vi "Verify Node GUID Matches Data Sharing Framework GUID.vi"(8 "error in":errorcluster, 11 "data sharing framework custom device in":T1 format="%.0x") -> (0 "error out":errorcluster, 3 "data sharing framework custom device out":T1 format="%.0x")   [LabVIEW 2021, in "Data Sharing Framework Custom Device Scripting.lvlib"]
uses:
  Data Sharing Framework Custom Device Scripting.lvlib
  <vilib>/NI VeriStand/Custom Device API/Custom Device Item Ref.ctl
  NationalInstruments.VeriStand.SystemDefinitionAPI
  Shared/DSF Shared.lvlib
  <vilib>/NI VeriStand/Custom Device API/Custom Device API.lvlib
panel:
  out "data sharing framework custom device node type":bool
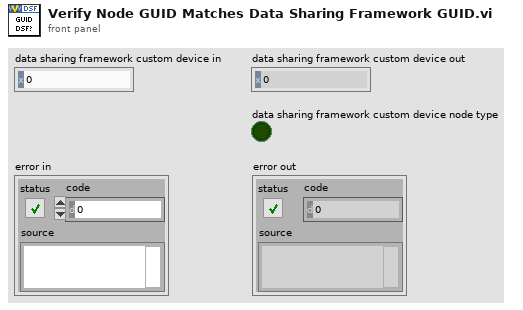
[diagram p1: front panel]
types:
  T1 = typedef "Custom Device API.lvlib/Custom Device Item Ref.ctl" = u64
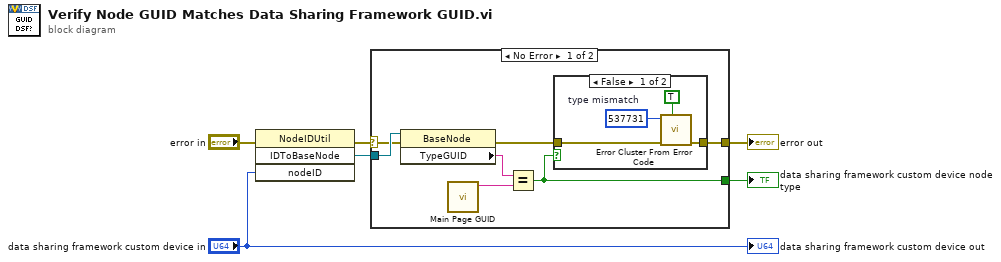
[diagram p0: block diagram]
diagram:
  n1 = invoke on="Invoke Node" class="NodeIDUtil" method="IDToBaseNode"(error in="error in", "nodeID"="data sharing framework custom device in") -> (error out=w5:errorcluster, "IDToBaseNode"=w6:refnum<k24>)  [unwired: 2 in, 2 out]
  n2 = case shown="No Error" w5 {
    selector: w5 -> [w12 w19]
    tunnel: w6 -> [w13 _]
    tunnel: [w8 w19] -> w4
    tunnel: [w9 _] -> w1
    frame No Error {
      n3 = property on="Property Node" class="BaseNode"(reference=w13, error in=w12) -> (error out=w7:errorcluster, "TypeGUID"=w11:string)  [unwired: 1 out]
      n4 = call "Main Page GUID.vi"() -> ("Main Page GUID"=w10:string)  [unwired: 11 in]
      n5 = Equal?(x=w11, y=w10) -> (x = y?=w9:bool)
      n6 = case shown="False" w9 {
        tunnel: [w14 w18] -> w8
        tunnel: w7 -> [w15 w18]
        frame False {
          w16 = 537731  # type mismatch
          n7 = call <vilib>:"Error Cluster From Error Code.vi"("show call chain? (False)"=TRUE, "error in (no error)"=w15, "error code (0)"=w16) -> ("error out"=w14:errorcluster)  [unwired: 6 in]
        }
        frame True {
        }
      }
    }
    frame Error {
    }
  }
  "error out" <- w4
  "data sharing framework custom device node type" <- w1
  "data sharing framework custom device out" <- "data sharing framework custom device in"
